vi "MU Read Register.vi"(8 "error in (no error)":errorcluster, 9 "count in":u32, 10 "address":u32, 11 "handle":u64) -> (0 "error out (no error)":errorcluster, 1 "count out":u32, 2 "values":u32[](array[numeric]), 3 "function return":u32)   [LabVIEW 2017, in "MU_3SL_interface.lvlib"]
uses:
  MU_3SL_interface.lvlib
  lib/MU_3SL_interface.dll
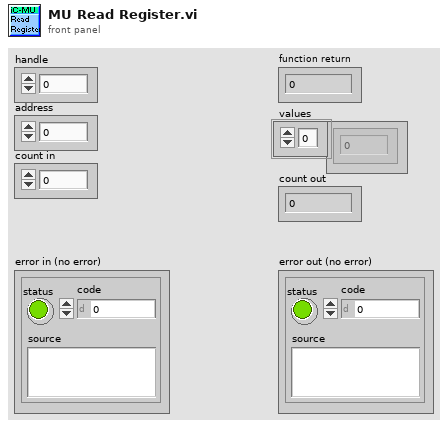
[diagram p1: front panel]
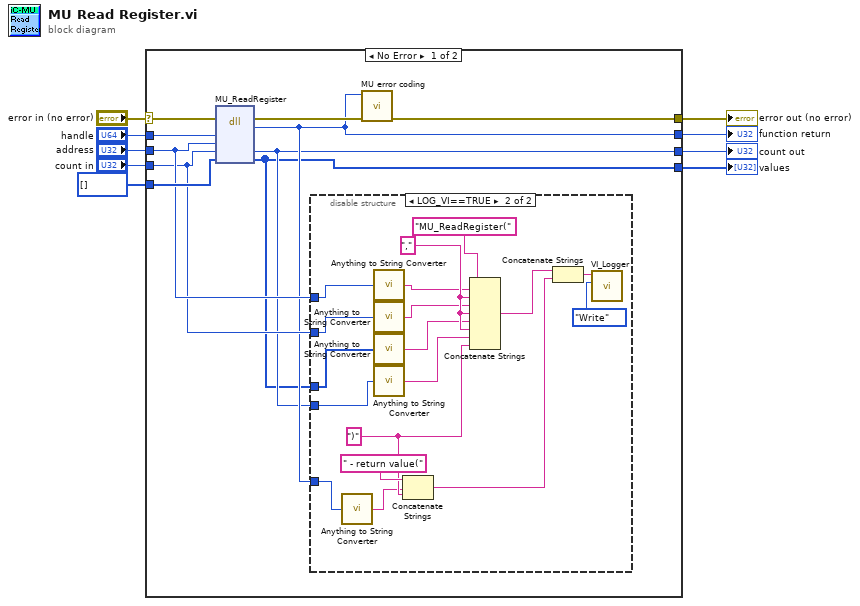
[diagram p0: block diagram]
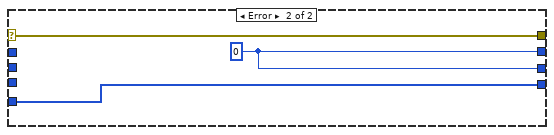
[diagram p3: hidden frame]
diagram:
  n1 = case shown="No Error" "error in (no error)" {
    selector: "error in (no error)" -> [w16 w40]
    tunnel: [w12 w38] -> w9
    tunnel: "handle" -> [w19 _]
    tunnel: "address" -> [w14 _]
    tunnel: "count in" -> [w13 _]
    tunnel: [w11 w38] -> w5
    tunnel: [w17 w40] -> w4
    tunnel: [w10 w39] -> w2
    tunnel: u32[] [] ("pulData") -> [w15 w39]
    frame No Error {
      n2 = dll-call lib="C:/Users/bes/AppData/Roaming/work/mu_9so/icsubmodules/soft_mu_3sl_master/lv_interface/lib/MU_3SL_interface**.*" fn="MU_ReadRegister"(error in=w16, "handle"=w19, "address"=w14, "count"=w13, "values"=w15) -> (error out=w18:errorcluster, "return type"=w12:u32, "count"=w11:u32, "values"=w10:u32[])  [unwired: 4 in, 1 out]
      n3 = disable-structure shown="LOG_VI==TRUE" {
        disable-tunnel: w12 -> [_ w25]
        disable-tunnel: w14 -> [_ w29]
        disable-tunnel: w13 -> [_ w28]
        disable-tunnel: w11 -> [_ w26]
        disable-tunnel: w10 -> [_ w27]
        frame condition #0 {
        }
        frame condition #1 (active) {
          w31 = ")" ("string")
          w32 = "," ("string")
          n4 = call "Anything to String Converter.vi"("anything"=w25) -> ("String"=w24:string)
          n5 = call "Anything to String Converter.vi"("anything"=w29) -> ("String"=w20:string)
          n6 = call "Anything to String Converter.vi"("anything"=w28) -> ("String"=w21:string)
          n7 = call "Anything to String Converter.vi"("anything"=w27) -> ("String"=w22:string)
          n8 = call "Anything to String Converter.vi"("anything"=w26) -> ("String"=w23:string)
          n9 = Concatenate Strings(" - return value(" ("string"), w24, w31) -> (w35:string)
          n10 = Concatenate Strings("MU_ReadRegister(" ("Info in"), w20, w32, w21, w32, w22, w32, w23, w31) -> (w30:string)
          n11 = Concatenate Strings(w30, w35) -> (w34:string)
          n12 = call "VI_Logger.vi"("Action (Read)"=enum16{"Write", "Read"}."Write", "Info in"=w34) -> ()  [unwired: 8 in, 2 out]
        }
      }
      n13 = call "MU error coding.vi"("error in (no error)"=w18, "function return in"=w12) -> ("error out"=w17:errorcluster)  [unwired: 9 in]
    }
    frame Error {
      w38 = u32 0 ("return type")
    }
  }
  "function return" <- w9
  "count out" <- w5
  "values" <- w2
  "error out (no error)" <- w4
